vi "salva_dista_arquivo.vi"() -> ()   [LabVIEW 2016]
uses:
  <vilib>/NXT/Subs/LVHSConnector.ctl
  <vilib>/NXT/LegoClasses/BrickReference/BrickReference.lvclass
panel:
  out "NXT/EV3 2":T1
  in  "NXT/EV3":T1
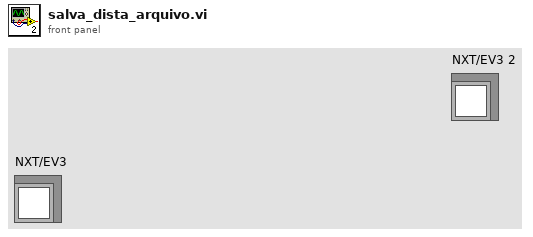
[diagram p1: front panel]
types:
  T1 = typedef "LVHSConnector.ctl" = refnum<class "BrickReference.lvclass">
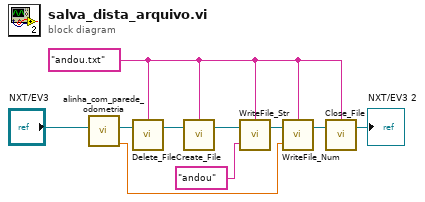
[diagram p0: block diagram]
diagram:
  w4 = "andou.txt" ("Filename")
  n1 = call "alinha_com_parede_odometria.vi"("NXT/EV3"="NXT/EV3") -> ("Numeric"=w1:dbl, "NXT/EV3 2"=w3:T1)  [unwired: 9 in]
  n2 = call <vilib>:"Delete_File.vi"("NXT/EV3"=w3, "Filename"=w4) -> ("NXT/EV3"=w9:T1)  [unwired: 2 in]
  n3 = call <vilib>:"Create_File.vi"("NXT/EV3"=w9, "Filename"=w4) -> ("NXT/EV3"=w8:T1)  [unwired: 2 in]
  n4 = call <vilib>:"WriteFile_Str.vi"("String"="andou", "NXT/EV3"=w8, "Filename"=w4) -> ("NXT/EV3"=w6:T1)  [unwired: 1 in]
  n5 = call <vilib>:"WriteFile_Num.vi"("Number"=w1, "NXT/EV3"=w6, "Filename"=w4) -> ("NXT/EV3"=w5:T1)  [unwired: 1 in]
  n6 = call <vilib>:"Close_File.vi"("NXT/EV3"=w5, "Filename"=w4) -> ("NXT/EV3"=→"NXT/EV3 2":T1)  [unwired: 2 in]
